vi "bboxsubvi.vi"(0 "Image":T1, 1 "size":dbl, 2 "def num":i32, 3 "array":dbl[][](array[numeric]), 4 "Drawing Mode (Frame)":u32(ring)=1 items=["Frame", "Fill"], 5 "error in":errorcluster) -> (14 "Image Out":T1, 19 "error out":errorcluster)   [LabVIEW 2019]
uses:
  <vilib>/vision/Image Controls.llb/IMAQ Image.ctl
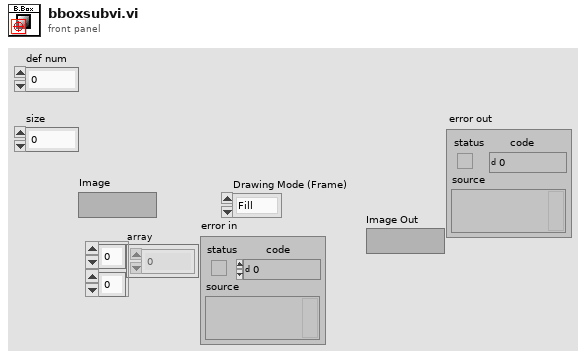
[diagram p1: front panel]
types:
  T1 = typedef "IMAQ Image.ctl" = refnum<image>
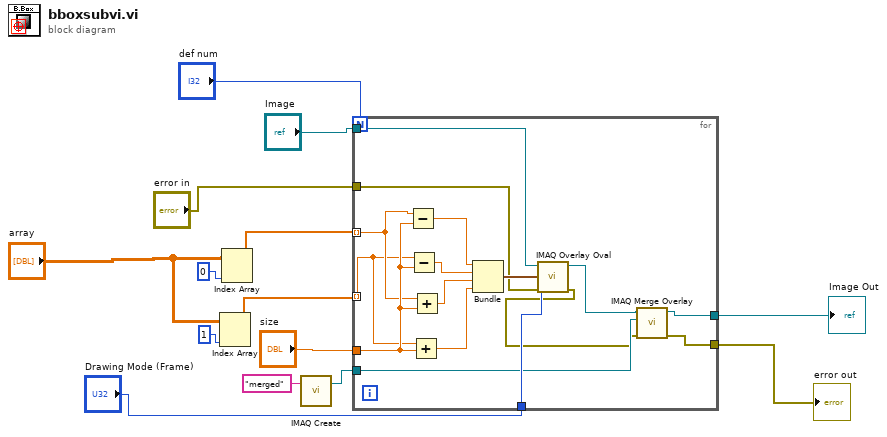
[diagram p0: block diagram]
diagram:
  n1 = Index Array(array="array", index (col)=1 ("index (row)")) -> (element=w13:dbl[])  [unwired: 1 in]
  n2 = Index Array(array="array", index (col)=0 ("index (row)")) -> (element=w14:dbl[])  [unwired: 1 in]
  n3 = call "IMAQ Create"("Image Name"="merged") -> ("New Image"=w1:T1)  [unwired: 4 in, 1 out]
  n4 = for {
    N: "def num" -> [_]
    tunnel: "size" -> [w30]
    tunnel: w14 -> [w26] mode=indexing
    tunnel: w13 -> [w25] mode=indexing
    tunnel: "Image" -> [w22]
    tunnel: "Drawing Mode (Frame)" -> [w21]
    tunnel: [w19] -> w9
    tunnel: [w18] -> w8
    tunnel: "error in" -> [w17]
    tunnel: w1 -> [w16]
    n5 = Subtract(x=w26, y=w30) -> (x-y=w29:dbl)
    n6 = Subtract(x=w25, y=w30) -> (x-y=w27:dbl)
    n7 = Add(x=w25, y=w30) -> (x+y=w23:dbl)
    n8 = Add(x=w26, y=w30) -> (x+y=w24:dbl)
    n9 = Bundle(w29, w27, w24, w23) -> (w28:cluster{dbl, dbl, dbl, dbl})  [unwired: 1 in]
    n10 = call "IMAQ Overlay Oval"("error in (no error)"=w17, "Drawing Mode (Frame)"=w21, "Bounding Rectangle"=w28, "Image"=w22) -> ("error out"=w15:errorcluster, "Image Out"=w20:T1)  [unwired: 6 in]
    n11 = call "IMAQ Merge Overlay"("error in (no error)"=w15, "Image Dst"=w16, "Image Src"=w20) -> ("error out"=w19:errorcluster, "Image Dst Out"=w18:T1)  [unwired: 7 in]
  }
  "Image Out" <- w8
  "error out" <- w9
